vi "pict set.vi"(10 "picture":picture, 11 "Sudoku in":refnum<class "Sudoku.lvclass">) -> (3 "Sudoku out":refnum<class "Sudoku.lvclass">)   [LabVIEW 2021, in "Sudoku.lvclass"]
uses:
  Sudoku.lvclass
  Sudoku.lvclass/Sudoku.ctl
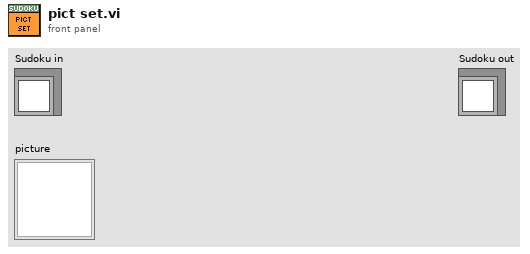
[diagram p1: front panel]
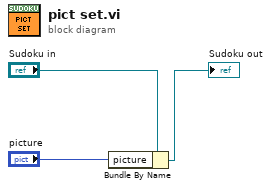
[diagram p0: block diagram]
diagram:
  n1 = Bundle By Name(cluster="Sudoku in", "picture"="picture") -> (→"Sudoku out":refnum<class "Sudoku.lvclass">)
